vi "UT__all.vi"   [LabVIEW 2017]
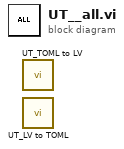
[diagram p0: block diagram]
diagram:
  n1 = call "UT_TOML to LV.vi"() -> ()  [unwired: 12 in]
  n2 = call "UT_LV to TOML.vi"() -> ()  [unwired: 12 in]
